vi "Current Features Popup.vi"(8 "error in":errorcluster, 10 "Strings []":string[](array[string]), 11 "Feature Type:":u16(ring) caption="New Feature Type:" items=["Corrugation", "Weld", "Crack", "Pit", "Joint", "wed", "Spalling", "Pitting", "Feature_2", "fetaure3", "Add New..."]) -> (0 "error out":errorcluster, 2 "Feature Type: 2":u16, 3 "Update?":bool)   [LabVIEW 2024]
uses:
  Buttons/Cancel.ctl
panel:
  in  "Feature Type Value":u16(ring) caption="New Feature Type:" items=["Corrugation", "Weld", "Crack", "Pit", "Joint", "wed", "Spalling", "Pitting", "Feature_2", "fetaure3", "Add New..."]
  in  "OK Button":bool
  in  "Cancel Button":T1
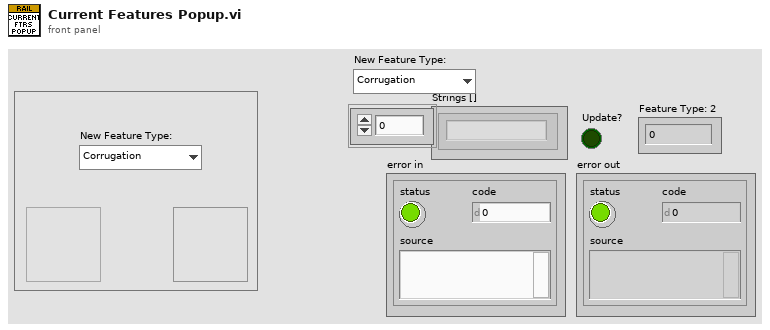
[diagram p1: front panel]
types:
  T1 = typedef "Cancel.ctl" = bool
  T2 = enum8{"Enabled", "Disabled", "Disabled and Grayed Out"}
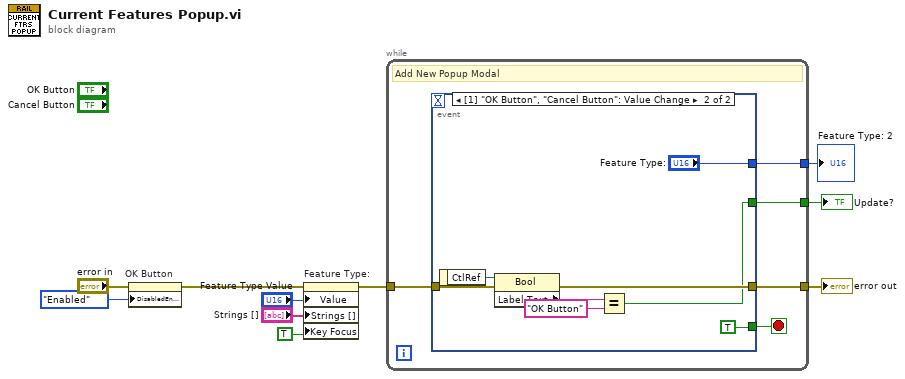
[diagram p0: block diagram]
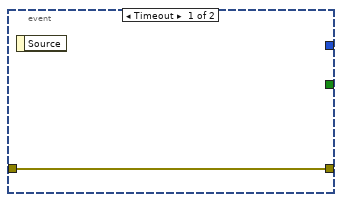
[diagram p2: hidden frame]
diagram:
  n1 = property on="OK Button" class="Bool"(error in="error in", "DisabledEnum"=T2."Enabled" ("Disabled")) -> (error out=w6:errorcluster)  [unwired: 1 in, 1 out]
  n2 = property on="Feature Type:" class="Ring (strict)"(error in=w6, "Value"="Feature Type Value", "Strings []"="Strings []", "Key Focus"=TRUE) -> (error out=w5:errorcluster)  [unwired: 1 in, 1 out]
  n3 = while {
    tunnel: w5 -> [w15]
    tunnel: [w14] -> w10
    tunnel: [w12] -> w7
    tunnel: [w11] -> w1
    stop <- w13 stop-if-true
    # "Add New Popup Modal"
    n4 = event shown="[1] \"OK Button\", \"Cancel Button\": Value Change" {
      selector: _ -> [_ _]
      dyn-events: _ -> [_ _]
      timeout: _ -> [_ _]
      tunnel: w15 -> [w16 w24]
      tunnel: [w16 w22] -> w14
      tunnel: [_ TRUE] -> w13
      tunnel: [_ w18] -> w12
      tunnel: [_ "Feature Type:"] -> w11
      event Timeout {
        n5 = event-data() -> ()  [unwired: 1 in, 1 out]
      }
      event "OK Button": Value Change {
        n6 = event-data() -> ("CtlRef"=w21:refnum<vi>)  [unwired: 1 in]
        n7 = property class="Bool"(reference=w21, error in=w24) -> (error out=w22:errorcluster, "Label.Text"=w20:string)  [unwired: 1 out]
        n8 = Equal?(x=w20, y="OK Button") -> (x = y?=w18:bool)
      }
    }
  }
  "error out" <- w10
  "Update?" <- w7
  "Feature Type: 2" <- w1
